vi "ITestSettings Raw Configuration to Specific Data Type.vi"(8 "error in (no error)":errorcluster, 10 "Raw Config Data":refnum<class "String Database.lvclass">[](array[class]), 11 "ITestSettings in":refnum<class "ITestSettings.lvclass">) -> (0 "error out":errorcluster, 3 "ITestSettings out":refnum<class "ITestSettings.lvclass">)   [LabVIEW 2016, in "ITestSettings.lvlib" / "ITestSettings.lvclass"]
uses:
  ITestSettings.lvclass
  Plugins/String Database.lvlibp/String Database.lvclass
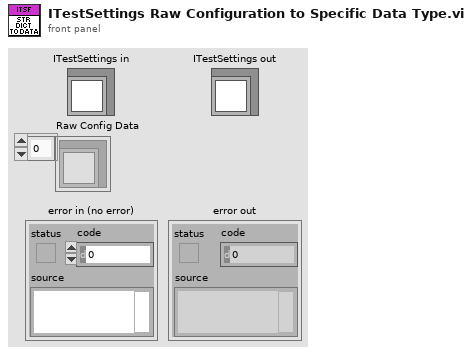
[diagram p1: front panel]
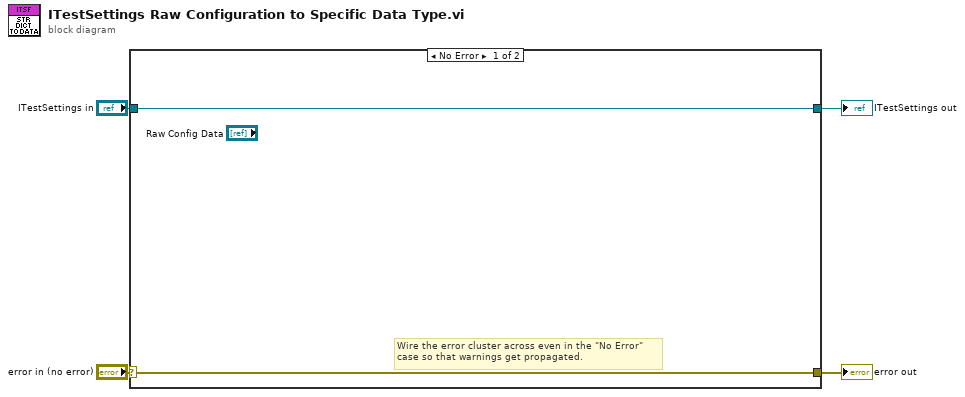
[diagram p0: block diagram]
diagram:
  n1 = case shown="No Error" "error in (no error)" {
    selector: "error in (no error)" -> [w5 w8]
    tunnel: [w5 w8] -> w3
    tunnel: [w6 w7] -> w1
    tunnel: "ITestSettings in" -> [w6 w7]
    frame No Error {
      # "Wire the error cluster across even in the \"No Error\"\ncase so that warnings get propagated."
    }
    frame Error {
    }
  }
  "error out" <- w3
  "ITestSettings out" <- w1
